vi "robotconperillas.vi"() -> ()   [LabVIEW 2016]
panel:
  out "XY Graph":cluster{dbl[], dbl[]}(graph)
  in  "L 3":dbl(slide) scale=0.0..3.0
  in  "L 2":dbl(slide) scale=0.0..3.0
  in  "L 1":dbl(slide) scale=0.0..3.0
  in  "T 3":dbl(knob) scale=0.0..360.0
  in  "T 2":dbl(knob) scale=0.0..360.0
  in  "T 1":dbl(knob) scale=0.0..360.0
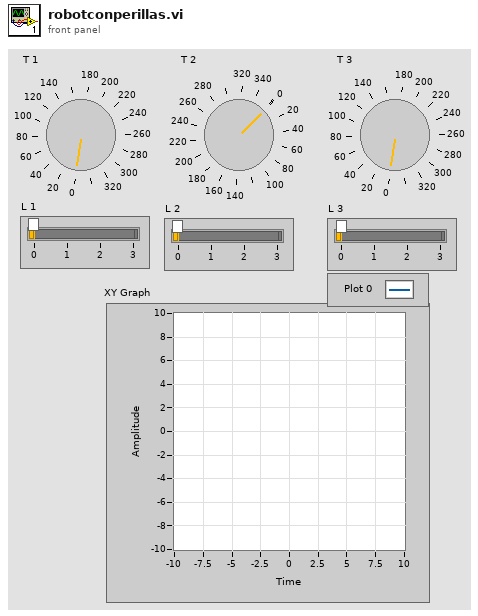
[diagram p1: front panel]
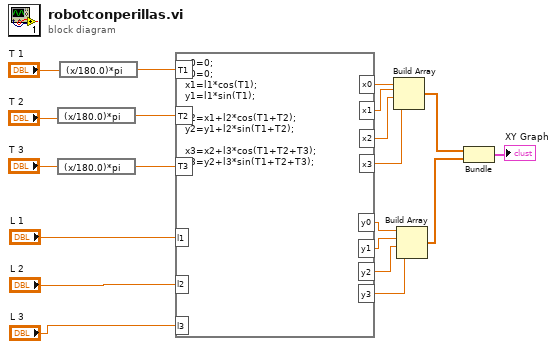
[diagram p0: block diagram]
diagram:
  n1 = expression code="(x/180.0)*pi" ("degrees to radians")("T 2") -> (w15:dbl)
  n2 = expression code="(x/180.0)*pi" ("degrees to radians")("T 3") -> (w7:dbl)
  n3 = expression code="(x/180.0)*pi" ("degrees to radians")("T 1") -> (w16:dbl)
  n4 = formula code="x0=0;\ny0=0;\nx1=l1*cos(T1);\ny1=l1*sin(T1);\n\nx2=x1+l2*cos(T1+T2);\ny2=y1+l2*sin(T1+T2);\n\nx3=x2+l3*cos(T1+T2+T3);\ny3=y2+l3*sin(T1+T2+T3);"("T1"=w16, "l1"="L 1", "T2"=w15, "T3"=w7, "l2"="L 2", "l3"="L 3") -> ("x0"=w14:dbl, "x1"=w13:dbl, "y0"=w12:dbl, "y1"=w11:dbl, "x2"=w6:dbl, "y2"=w5:dbl, "y3"=w2:dbl, "x3"=w1:dbl)
  n5 = Build Array(w14, w13, w6, w1) -> (w10:dbl[])
  n6 = Build Array(w12, w11, w5, w2) -> (w9:dbl[])
  n7 = Bundle(w10, w9) -> (→"XY Graph":cluster{dbl[], dbl[]})  [unwired: 1 in]
